vi "_Parse SEM Limit Check Result.vi"(8 "error in (no error)":errorcluster, 10 "Input String":string, 11 "VISA resource name":refnum<visa-resource-name>) -> (0 "error out":errorcluster, 1 "Measurement Result":T1 {"Out Of Tolerance" format="%^.3e"}, 2 "Reliability":i32, 3 "VISA resource name out":refnum<visa-resource-name>)   [LabVIEW 2020, in "Rohde&Schwarz CMXP NR FR2 Measurement.lvlib"]
uses:
  <instrlib>/Rohde&Schwarz CMXP NR FR2 Measurement/Rohde&Schwarz CMXP NR FR2 Measurement.lvlib
  <instrlib>/Rohde&Schwarz CMXP NR FR2 Measurement/Private/rsidr_core.llb/rsidr_core.lvlib
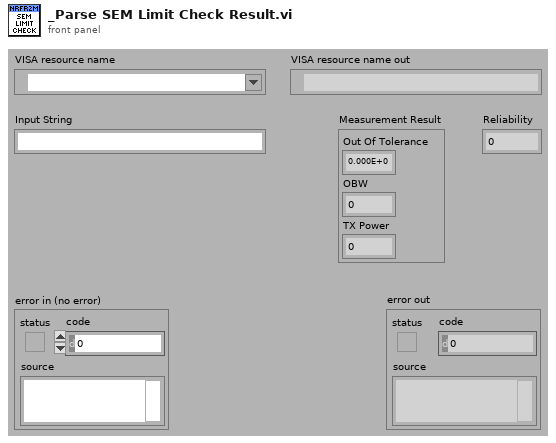
[diagram p1: front panel]
types:
  T1 = cluster{"Out Of Tolerance":dbl, "OBW":i32, "TX Power":i32}
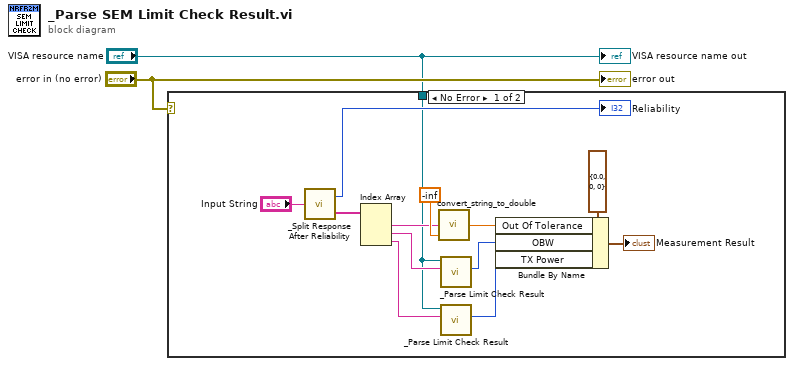
[diagram p0: block diagram]
diagram:
  n1 = case shown="No Error" "error in (no error)" {
    tunnel: "VISA resource name" -> [w3 _]
    frame No Error {
      n2 = call <instrlib>:"_Split Response After Reliability.vi"("Input String"="Input String") -> ("Response out"=w8:string[], "Reliability out"=→"Reliability":i32)
      n3 = Index Array(array=w8) -> (element #1=w7:string, element #2=w6:string, element #3=w5:string)  [unwired: 3 in]
      n4 = call <instrlib>:"convert_string_to_double.vi"("default (0)"=-inf, "String in"=w7) -> ("double value out"=w13:dbl)  [unwired: 3 in]
      n5 = call <instrlib>:"_Parse Limit Check Result.vi"("String Value In"=w6, "VISA resource name"=w3) -> ("Limit Check Value"=w12:i32)  [unwired: 7 in, 2 out]
      n6 = call <instrlib>:"_Parse Limit Check Result.vi"("String Value In"=w5, "VISA resource name"=w3) -> ("Limit Check Value"=w11:i32)  [unwired: 7 in, 2 out]
      n7 = Bundle By Name(cluster=T1 {"Out Of Tolerance"=0.0, "OBW"=0, "TX Power"=0} ("Measurement Result"), "Out Of Tolerance"=w13, "OBW"=w12, "TX Power"=w11) -> (→"Measurement Result":T1)
    }
    frame Error {
    }
  }
  "error out" <- "error in (no error)"
  "VISA resource name out" <- "VISA resource name"
